vi "Actor Core.vi"(8 "error in":errorcluster, 11 "Platform in":refnum<class "Platform.lvclass">) -> (0 "error out":errorcluster, 3 "Actor out":refnum<class "Actor.lvclass">)   [LabVIEW 2019, in "Platform.lvlib" / "Platform.lvclass"]
doc: "(<B>Filename</B>: Actor Framework.lvlib:Actor.lvclass:Actor Core.vi)\n\nReceives messages to the actor, reacts to them, and initiates any error handling that may shut the actor down.\n\nDescendant classes may override this VI to append parallel tasks for the actor to complete while it handles messages. Overrides use the Call Parent Method node."
uses:
  Platform.lvclass
  C:/Program Files (x86)/National Instruments/LabVIEW 2019/vi.lib/MGI/Panel Manager/Panel Actor/Panel Actor/Panel Actor.lvclass
  C:/Program Files (x86)/National Instruments/LabVIEW 2019/vi.lib/ActorFramework/Actor/Actor.lvclass
  <vilib>/ActorFramework/Actor/Actor.lvclass
  Platform.lvclass/Platform.ctl
  <vilib>/ActorFramework/Message Enqueuer/Message Enqueuer.lvclass/Message Enqueuer.ctl
  Sequence/Sequence Messages/Load Seq Msg/Load Seq Msg.lvclass/Load Seq Msg.ctl
  Sequence/Sequence Messages/Update Seq Msg/Update Seq Msg.lvclass/Update Seq Msg.ctl
  <vilib>/ActorFramework/Actor/Actor.lvclass/Actor.ctl
  Timer/Timer Messages/Start Timer Msg/Start Timer Msg.lvclass/Start Timer Msg.ctl
  Platform Messages/Run Msg/PF Commands Msg.lvclass/PF Commands Msg.ctl
  <vilib>/ActorFramework/Message Enqueuer/Enqueue.vi
  Timer/Timer Messages/Read Timer Msg/Read Timer Msg.lvclass
  C:/Program Files (x86)/National Instruments/LabVIEW 2019/vi.lib/ActorFramework/Message/Message.lvclass
  Sequence/Sequence Messages/Load Seq Msg/Load Seq Msg.lvclass
  Sequence/Sequence Messages/Update Seq Msg/Update Seq Msg.lvclass
  Timer/Timer Messages/Pause Timer Msg/Pause Timer Msg.lvclass
  Timer/Timer Messages/Resume Timer Msg/Resume Timer Msg.lvclass
  Timer/Timer Messages/Start Timer Msg/Start Timer Msg.lvclass
  Platform Messages/Run Msg/PF Commands Msg.lvclass
  <vilib>/ActorFramework/Stop Msg/Stop Msg.lvclass
  <userlib>/_MGI/Application Control/MGI Get Value/MGI Get Value (BOOL).vi
  <userlib>/_MGI/Application Control/MGI Get Value/MGI Get Value (I32).vi
  <vilib>/ActorFramework/Message Priority Queue/Priority Enqueue.vi
  <userlib>/_MGI/Application Control/MGI Gray if/MGI Gray if False.vi
  <vilib>/MGI/Panel Manager/Panel Actor/Panel Actor/Panel Actor.lvclass
panel:
  in  "Sequence":T1(array[cluster]) {"Duration" format="%<%H:%M:%S>t"}
  in  "Clear":bool
  in  "Save":bool
  in  "Sequence File Path":path=path "C:/Working Copy/trunk/Modified Cobra Jung/Cobra/Power Pattern Configuration/TTV.ini" caption="Path"
  out "Saving":bool
  out "Mini Graph":u32[](graph)
  in  "Run":bool
  out "Current Step":i32=1 caption="Step"
  out "Current Iteration":i32=1 caption="Iteration"
  in  "Reset Test":bool
  out "Elapsed Time":dbl caption="Time(sec)" format="%<%H:%M:%S>t"
  out "Test Graph":dbl[][](graph)
  in  "Iteration":i32=2
  out "Save File Path":path caption="Path"
  # "Step"
  # "Duration"
  # "Amplitute"
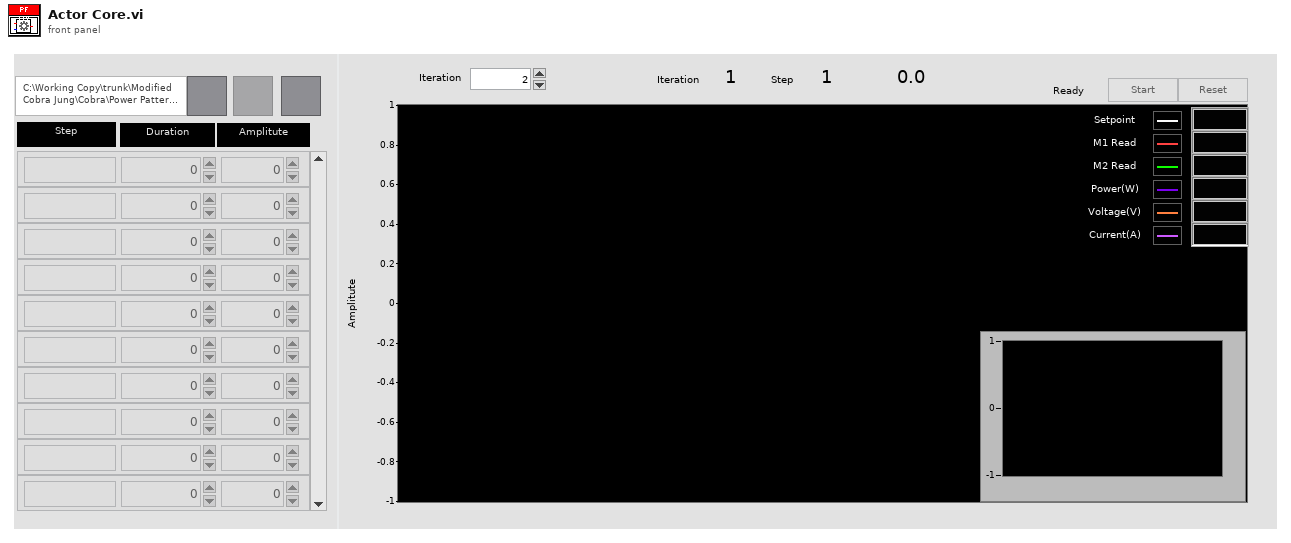
[diagram p1: front panel]
types:
  T1 = cluster{"Duration":i32, "Value":u32, "Name":string}[]
  T2 = enum32{"Invalid", "Standard", "Closed", "Hidden", "Minimized", "Maximized"}
  T3 = cluster{"Event Registration Refnum":refnum<event-registration>, "Pnl Actor":refnum<event-registration>}
  T4 = enum8{"Enabled", "Disabled", "Disabled and Grayed Out"}
  T5 = cluster{"Duration":i32, "Value":u32, "Name":string}
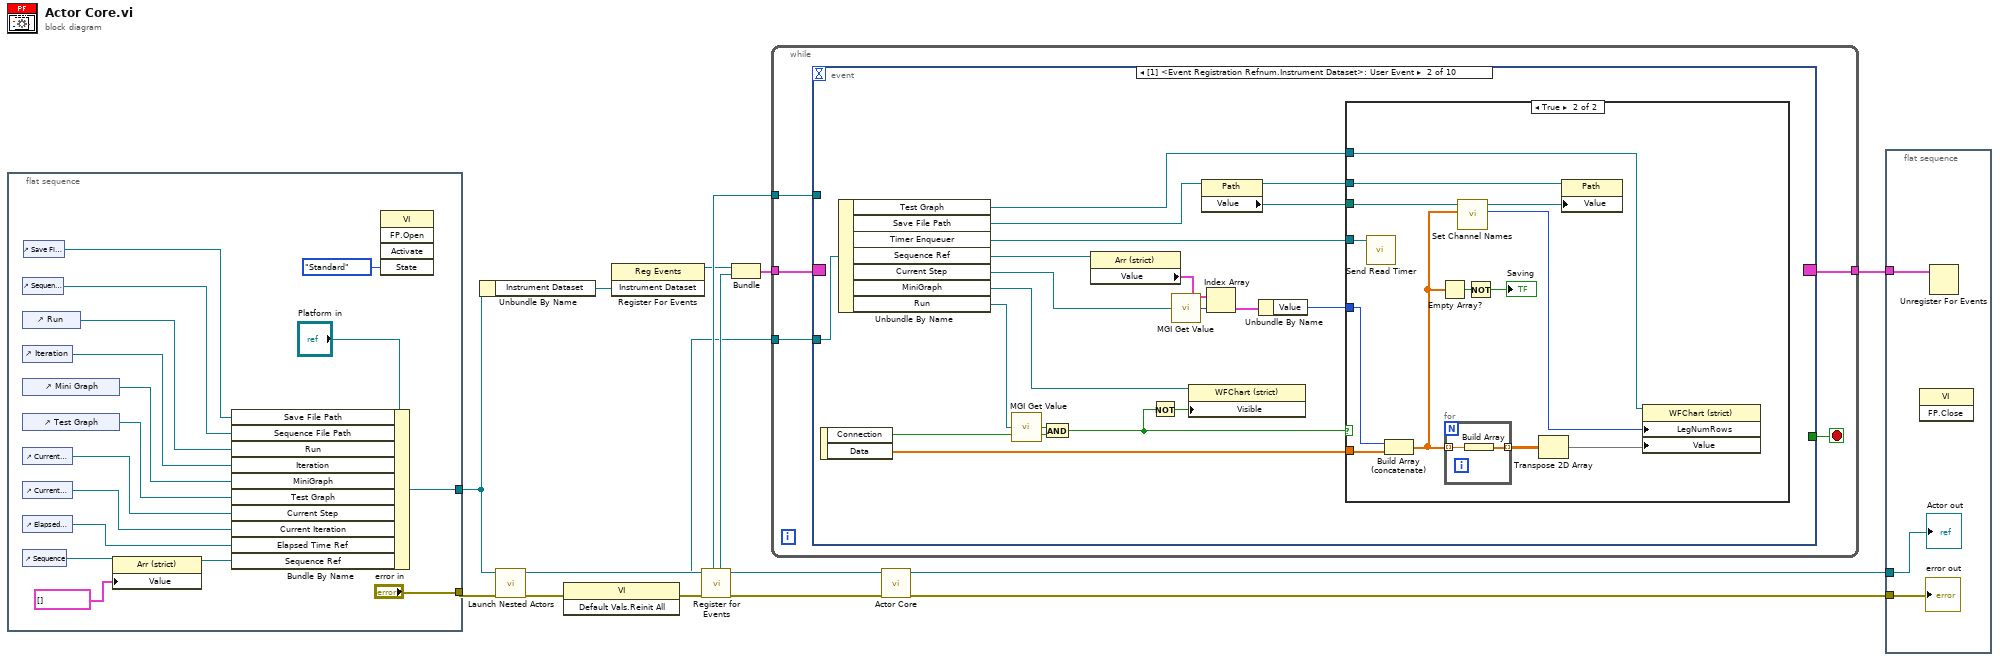
[diagram p0: block diagram]
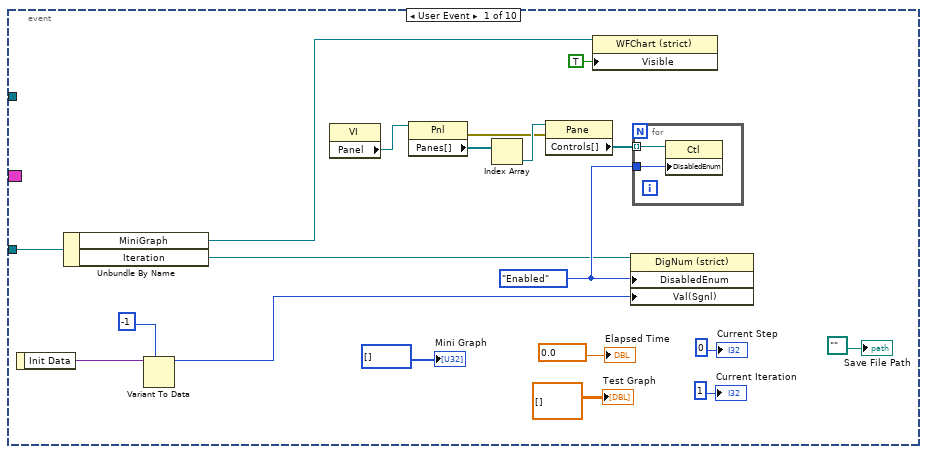
[diagram p2: hidden frame]
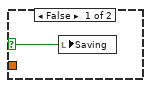
[diagram p3: hidden frame]
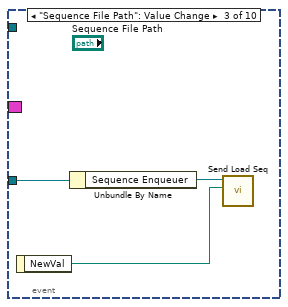
[diagram p4: hidden frame]
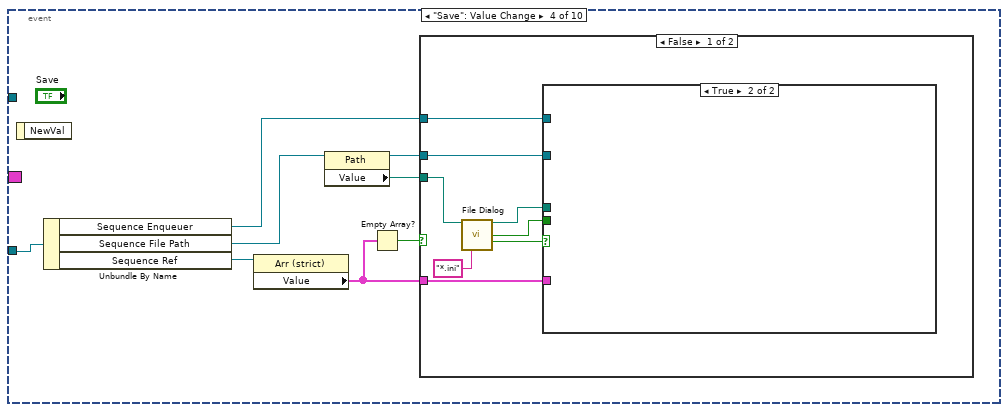
[diagram p5: hidden frame]
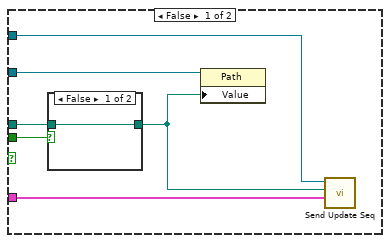
[diagram p6: hidden frame]
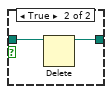
[diagram p7: hidden frame]
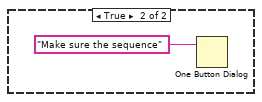
[diagram p8: hidden frame]
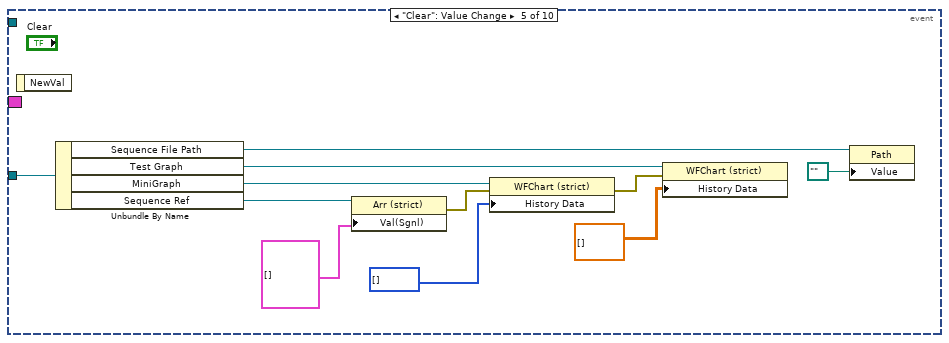
[diagram p9: hidden frame]
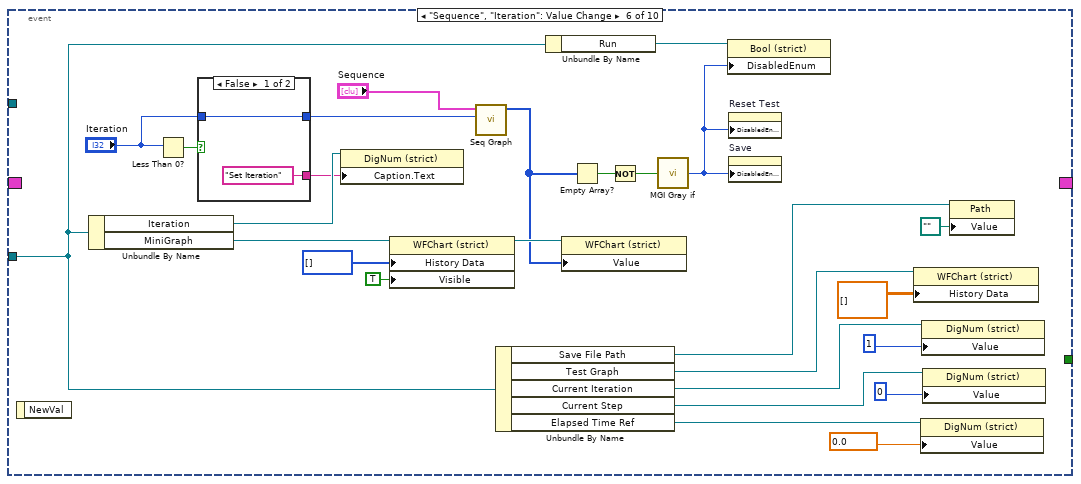
[diagram p10: hidden frame]
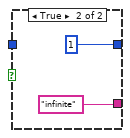
[diagram p11: hidden frame]
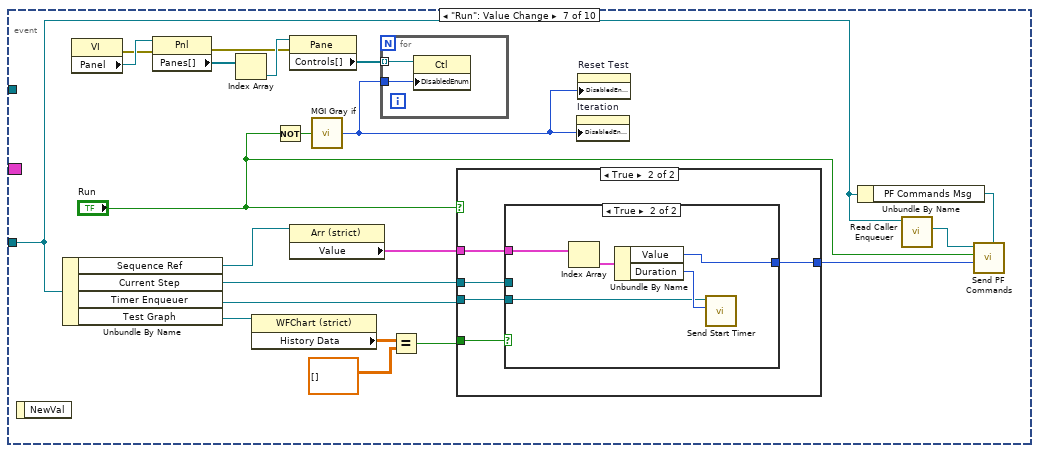
[diagram p12: hidden frame]
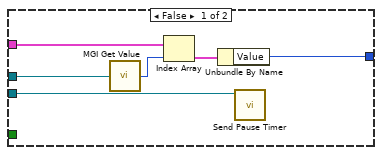
[diagram p13: hidden frame]
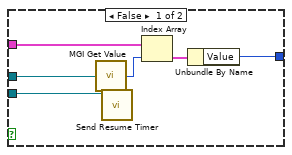
[diagram p14: hidden frame]
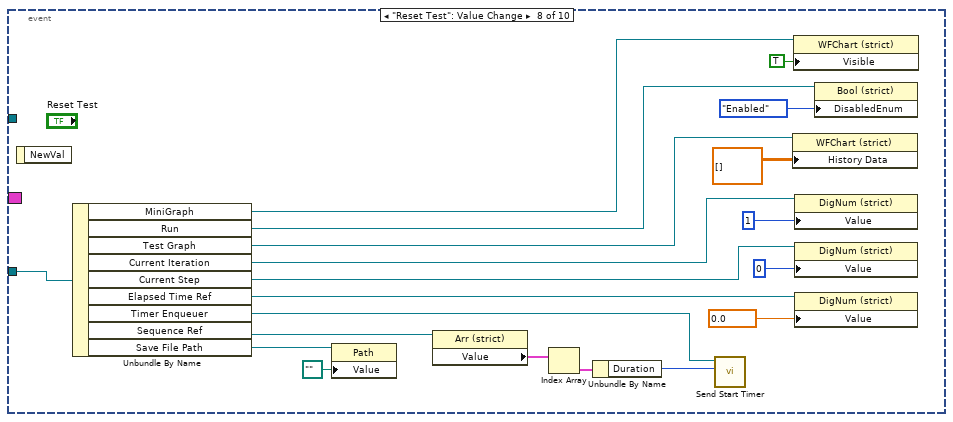
[diagram p15: hidden frame]
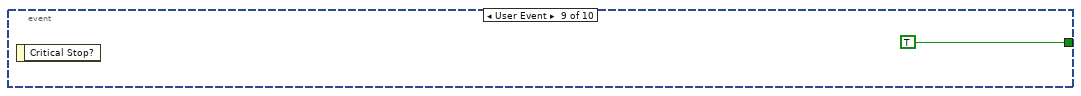
[diagram p16: hidden frame]
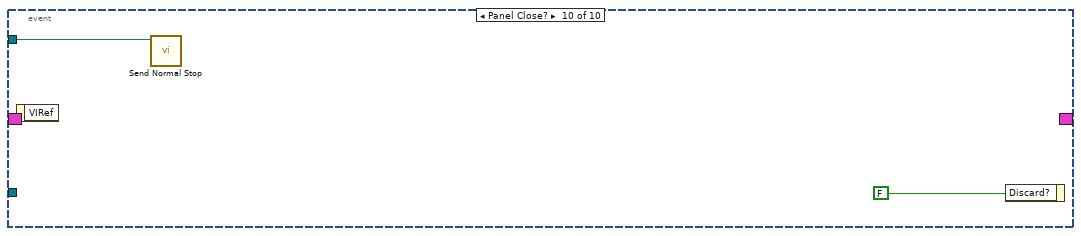
[diagram p17: hidden frame]
diagram:
  n1 = flat-sequence {
    tunnel: ["error in"] -> w5
    tunnel: [w24] -> w4
    frame #0 {
      n2 = control-ref of="Sequence File Path"() -> (w17:refnum<vi>)
      n3 = control-ref of="Run"() -> (w23:refnum<vi>)
      n4 = control-ref of="Iteration"() -> (w25:refnum<vi>)
      n5 = control-ref of="Mini Graph"() -> (w22:refnum<vi>)
      n6 = control-ref of="Test Graph"() -> (w21:refnum<vi>)
      n7 = control-ref of="Current Step"() -> (w28:refnum<vi>)
      n8 = control-ref of="Current Iteration"() -> (w27:refnum<vi>)
      n9 = control-ref of="Elapsed Time"() -> (w29:refnum<vi>)
      n10 = control-ref of="Sequence"() -> (w19:refnum<vi>)
      n11 = control-ref of="Save File Path"() -> (w16:refnum<vi>)
      n12 = property class="Arr (strict)"(reference=w19, "Value"=T1 [] ("Sequence")) -> (reference out=w18:refnum<vi>)  [unwired: 1 in, 1 out]
      n13 = Bundle By Name(cluster="Platform in", "Save File Path"=w16, "Sequence File Path"=w17, "Run"=w23, "Iteration"=w25, "MiniGraph"=w22, "Test Graph"=w21, "Current Step"=w28, "Current Iteration"=w27, "Elapsed Time Ref"=w29, "Sequence Ref"=w18) -> (w24:refnum<class "Platform.lvclass">)
      n14 = invoke class="VI" method="FP.Open"("State"=T2."Standard") -> ()  [unwired: 4 in, 5 out]
    }
  }
  n15 = Unbundle By Name(w4) -> ("Instrument Dataset"=w9:refnum<user-event>)
  n16 = call-dynamic "Launch Nested Actors.vi"("error in"=w5, "Platform in"=w4) -> ("error out"=w3:errorcluster, "Platform out"=w11:refnum<class "Platform.lvclass">)  [unwired: 8 in]
  n17 = invoke class="VI" method="Default Vals.Reinit All"(error in=w3) -> (error out=w2:errorcluster)  [unwired: 2 in, 2 out]
  n18 = register-events(w9) -> (reference out=w6:refnum<event-registration>)  [unwired: 2 in, 1 out]
  n19 = call <vilib>:"Register for Events.vi"("Error In"=w2, "Panel Actor in"=w11) -> ("Error Out"=w12:errorcluster, "Panel Actor out"=w1:refnum<class "Platform.lvclass">, "Pnl Actor"=w8:refnum<event-registration>, "Self Enqueuer"=w10:refnum<class "Message Enqueuer.lvclass">)  [unwired: 6 in]
  n20 = Bundle("Event Registration Refnum"=w6, "Pnl Actor"=w8) -> (w7:T3)  [unwired: 1 in]
  n21 = while {
    tunnel: w7 -> [w36]
    tunnel: [w34] -> w13
    tunnel: w10 -> [w33]
    tunnel: w1 -> [w32]
    stop <- w35 stop-if-true
    n22 = event shown="[1] <Event Registration Refnum.Instrument Dataset>: User Event" {
      selector: w36 -> [_ _ _ _ _ _ _ _ _ _]
      dyn-events: [_ _ _ _ _ _ _ _ _ _] -> w34
      timeout: _ -> [_ _ _ _ _ _ _ _ _ _]
      tunnel: [_ _ _ _ _ _ _ _ TRUE _] -> w35
      tunnel: w33 -> [_ _ _ _ _ _ _ _ _ w229]
      tunnel: w32 -> [w54 w73 w94 w103 w132 w143 w167 w225 _ _]
      event User Event {
        w47 = T4."Enabled" ("Disabled")
        n23 = event-data() -> ("Init Data"=w55:variant)  [unwired: 1 in]
        n24 = Unbundle By Name(w54) -> ("MiniGraph"=w44:refnum<vi>, "Iteration"=w46:refnum<vi>)
        n25 = Variant To Data(type=-1 ("Value (Signaling)"), Variant=w55) -> (data=w37:i32)  [unwired: 1 in, 1 out]
        n26 = property class="VI"() -> ("Panel"=w48:refnum<vi>)  [unwired: 2 in, 2 out]
        n27 = property class="Pnl"(reference=w48) -> (error out=w49:errorcluster, "Panes[]"=w52:refnum<vi>[])  [unwired: 1 in, 1 out]
        n28 = Index Array(array=w52) -> (element=w51:refnum<vi>)  [unwired: 1 in]
        n29 = property class="Pane"(reference=w51, error in=w49) -> ("Controls[]"=w50:refnum<vi>[])  [unwired: 2 out]
        n30 = property class="WFChart (strict)"(reference=w44, "Visible"=TRUE) -> ()  [unwired: 1 in, 2 out]
        n31 = property class="DigNum (strict)"(reference=w46, "DisabledEnum"=w47, "Val(Sgnl)"=w37) -> ()  [unwired: 1 in, 2 out]
        n32 = for {
          tunnel: w50 -> [w57] mode=indexing
          tunnel: w47 -> [w56]
          n33 = property class="Ctl"(reference=w57, "DisabledEnum"=w56) -> ()  [unwired: 1 in, 2 out]
        }
        "Current Step" <- 0 ("Current Step")
        "Current Iteration" <- 1 ("Current Iteration")
        "Mini Graph" <- u32[] [] ("Test Graph")
        "Elapsed Time" <- 0.0 ("Time")
        "Test Graph" <- dbl[][] [] ("Test Graph")
        "Save File Path" <- path "" ("Save File Path")
      }
      event User Event {
        n34 = event-data() -> ("Connection"=w68:bool, "Data"=w76:dbl[])  [unwired: 1 in]
        n35 = Unbundle By Name(w73) -> ("Test Graph"=w58:refnum<vi>, "Save File Path"=w63:refnum<vi>, "Timer Enqueuer"=w67:refnum<class "Message Enqueuer.lvclass">, "Sequence Ref"=w75:refnum<vi>, "Current Step"=w72:refnum<vi>, "MiniGraph"=w61:refnum<vi>, "Run"=w64:refnum<vi>)
        n36 = call-poly <userlib>:"MGI Get Value.vi"("Ref"=w64) -> ("Value"=w65:bool)
        n37 = And(x=w65, y=w68) -> (x .and. y?=w60:bool)
        n38 = property class="Arr (strict)"(reference=w75) -> ("Value"=w74:T1)  [unwired: 1 in, 2 out]
        n39 = Not(x=w60) -> (.not. x?=w66:bool)
        n40 = call-poly <userlib>:"MGI Get Value.vi"("Ref"=w72) -> ("Value"=w71:i32)
        n41 = property class="WFChart (strict)"(reference=w61, "Visible"=w66) -> ()  [unwired: 1 in, 2 out]
        n42 = property class="Path"(reference=w63) -> (reference out=w59:refnum<vi>, "Value"=w62:path)  [unwired: 1 in, 1 out]
        n43 = Index Array(array=w74, index=w71) -> (element=w70:T5)
        n44 = Unbundle By Name(w70) -> ("Value"=w69:u32)
        n45 = case shown="True" w60 {
          selector: w60 -> [w77 _]
          tunnel: w76 -> [_ w80]
          tunnel: w67 -> [_ w90]
          tunnel: w69 -> [_ w81]
          tunnel: w62 -> [_ w85]
          tunnel: w59 -> [_ w89]
          tunnel: w58 -> [_ w87]
          frame False {
            n46 = local write "Saving"(w77) -> ()
          }
          frame True {
            n47 = call "Send Read Timer.vi"("Message Enqueuer"=w90) -> ()  [unwired: 9 in, 2 out]
            n48 = Build Array (concatenate)(w81, w80) -> (w79:dbl[])
            n49 = Empty Array?(array=w79) -> (empty?=w88:bool)
            n50 = for {
              tunnel: w79 -> [w91] mode=indexing
              tunnel: [w92] -> w86 mode=indexing
              n51 = Build Array(w91) -> (w92:dbl[])
            }
            n52 = call "Set Channel Names.vi"("Data"=w79, "file path (dialog if empty)"=w85) -> ("Channel Length"=w83:i32, "new file path (Not A Path if cancelled)"=w84:path)  [unwired: 8 in]
            n53 = Not(x=w88) -> (.not. x?=→"Saving":bool)
            n54 = Transpose 2D Array(2D array=w86) -> (transposed array=w82:dbl[][])
            n55 = property class="Path"(reference=w89, "Value"=w84) -> ()  [unwired: 1 in, 2 out]
            n56 = property class="WFChart (strict)"(reference=w87, "LegNumRows"=w83, "Value"=w82) -> ()  [unwired: 1 in, 2 out]
          }
        }
      }
      event "Sequence File Path": Value Change {
        n57 = event-data() -> ("NewVal"=w95:path)  [unwired: 1 in]
        n58 = Unbundle By Name(w94) -> ("Sequence Enqueuer"=w93:refnum<class "Message Enqueuer.lvclass">)
        n59 = call "Send Load Seq.vi"("Seq file path"=w95, "Message Enqueuer"=w93) -> ()  [unwired: 8 in, 2 out]
      }
      event "Save": Value Change {
        n60 = event-data() -> ()  [unwired: 1 in, 1 out]
        n61 = Unbundle By Name(w103) -> ("Sequence Enqueuer"=w97:refnum<class "Message Enqueuer.lvclass">, "Sequence File Path"=w99:refnum<vi>, "Sequence Ref"=w102:refnum<vi>)
        n62 = property class="Arr (strict)"(reference=w102) -> ("Value"=w101:T1)  [unwired: 1 in, 2 out]
        n63 = property class="Path"(reference=w99) -> (reference out=w96:refnum<vi>, "Value"=w98:path)  [unwired: 1 in, 1 out]
        n64 = Empty Array?(array=w101) -> (empty?=w100:bool)
        n65 = case shown="False" w100 {
          tunnel: w97 -> [w107 _]
          tunnel: w101 -> [w106 _]
          tunnel: w98 -> [w111 _]
          tunnel: w96 -> [w104 _]
          frame False {
            n66 = call "File Dialog"("start path"=w111, "pattern (all files)"="*.ini") -> ("selected path"=w108:path, "exists"=w109:bool, "cancelled"=w105:bool)  [unwired: 10 in, 1 out]
            n67 = case shown="True" w105 {
              tunnel: w109 -> [w117 _]
              tunnel: w108 -> [w116 _]
              tunnel: w107 -> [w115 _]
              tunnel: w106 -> [w114 _]
              tunnel: w104 -> [w112 _]
              frame False {
                n68 = case shown="False" w117 {
                  tunnel: w116 -> [w118 w120]
                  tunnel: [w118 w119] -> w113
                  frame False {
                  }
                  frame True {
                    n69 = Delete(path (use dialog)=w120) -> (deleted path=w119:path)  [unwired: 4 in, 2 out]
                  }
                }
                n70 = property class="Path"(reference=w112, "Value"=w113) -> ()  [unwired: 1 in, 2 out]
                n71 = call "Send Update Seq.vi"("Sequence"=w114, "file path"=w113, "Message Enqueuer"=w115) -> ()  [unwired: 7 in, 2 out]
              }
              frame True {
              }
            }
          }
          frame True {
            n72 = One Button Dialog(message="Make sure the sequence") -> ()  [unwired: 1 in, 1 out]
          }
        }
      }
      event "Clear": Value Change {
        n73 = event-data() -> ()  [unwired: 1 in, 1 out]
        n74 = Unbundle By Name(w132) -> ("Sequence File Path"=w123:refnum<vi>, "Test Graph"=w131:refnum<vi>, "MiniGraph"=w130:refnum<vi>, "Sequence Ref"=w128:refnum<vi>)
        n75 = property class="Arr (strict)"(reference=w128, "Val(Sgnl)"=T1 [] ("Value (Signaling)")) -> (error out=w126:errorcluster)  [unwired: 1 in, 1 out]
        n76 = property class="WFChart (strict)"(reference=w130, error in=w126, "History Data"=u32[] []) -> (error out=w125:errorcluster)  [unwired: 1 out]
        n77 = property class="WFChart (strict)"(reference=w131, error in=w125, "History Data"=dbl[][] [] ("Test Graph")) -> ()  [unwired: 2 out]
        n78 = property class="Path"(reference=w123, "Value"=path "" ("Sequence File Path")) -> ()  [unwired: 1 in, 2 out]
      }
      event "Sequence", "Iteration": Value Change {
        n79 = event-data() -> ()  [unwired: 1 in, 1 out]
        n80 = Unbundle By Name(w143) -> ("Iteration"=w151:refnum<vi>, "MiniGraph"=w154:refnum<vi>)
        n81 = Less Than 0?(x="Iteration") -> (x < 0?=w156:bool)
        n82 = case shown="False" w156 {
          tunnel: "Iteration" -> [w160 _]
          tunnel: [w160 1 ("t")] -> w157
          tunnel: ["Set Iteration" ("Inifinite") "infinite" ("Inifinite")] -> w150
          frame False {
          }
          frame True {
          }
        }
        n83 = property class="DigNum (strict)"(reference=w151, "Caption.Text"=w150) -> ()  [unwired: 1 in, 2 out]
        n84 = property class="WFChart (strict)"(reference=w154, "History Data"=u32[] [], "Visible"=TRUE) -> (reference out=w152:refnum<vi>)  [unwired: 1 in, 1 out]
        n85 = call "Seq Graph.vi"("Iteration"=w157, "Sequence"="Sequence") -> ("Waveform"=w141:u32[])  [unwired: 8 in, 1 out]
        n86 = Unbundle By Name(w143) -> ("Save File Path"=w134:refnum<vi>, "Test Graph"=w140:refnum<vi>, "Current Iteration"=w147:refnum<vi>, "Current Step"=w148:refnum<vi>, "Elapsed Time Ref"=w149:refnum<vi>)
        n87 = Unbundle By Name(w143) -> ("Run"=w142:refnum<vi>)
        n88 = property class="WFChart (strict)"(reference=w152, "Value"=w141) -> ()  [unwired: 1 in, 2 out]
        n89 = Empty Array?(array=w141) -> (empty?=w138:bool)
        n90 = Not(x=w138) -> (.not. x?=w137:bool)
        n91 = call-poly <userlib>:"MGI Gray if.vi"("Boolean"=w137) -> ("Disabled"=w136:T4)
        n92 = property class="Bool (strict)"(reference=w142, "DisabledEnum"=w136) -> ()  [unwired: 1 in, 2 out]
        n93 = property on="Reset Test" class="Bool"("DisabledEnum"=w136) -> ()  [unwired: 2 in, 2 out]
        n94 = property on="Save" class="Bool"("DisabledEnum"=w136) -> ()  [unwired: 2 in, 2 out]
        n95 = property class="WFChart (strict)"(reference=w140, "History Data"=dbl[][] [] ("Test Graph")) -> ()  [unwired: 1 in, 2 out]
        n96 = property class="DigNum (strict)"(reference=w149, "Value"=0.0 ("Time")) -> ()  [unwired: 1 in, 2 out]
        n97 = property class="DigNum (strict)"(reference=w147, "Value"=1) -> ()  [unwired: 1 in, 2 out]
        n98 = property class="DigNum (strict)"(reference=w148, "Value"=0) -> ()  [unwired: 1 in, 2 out]
        n99 = property class="Path"(reference=w134, "Value"=path "") -> ()  [unwired: 1 in, 2 out]
      }
      event "Run": Value Change {
        n100 = event-data() -> ()  [unwired: 1 in, 1 out]
        n101 = Unbundle By Name(w167) -> ("Sequence Ref"=w168:refnum<vi>, "Current Step"=w172:refnum<vi>, "Timer Enqueuer"=w183:refnum<class "Message Enqueuer.lvclass">, "Test Graph"=w171:refnum<vi>)
        n102 = property class="VI"() -> (error out=w178:errorcluster, "Panel"=w182:refnum<vi>)  [unwired: 2 in, 1 out]
        n103 = property class="Pnl"(reference=w182, error in=w178) -> (error out=w177:errorcluster, "Panes[]"=w181:refnum<vi>[])  [unwired: 1 out]
        n104 = Index Array(array=w181) -> (element=w180:refnum<vi>)  [unwired: 1 in]
        n105 = property class="WFChart (strict)"(reference=w171) -> ("History Data"=w170:dbl[][])  [unwired: 1 in, 2 out]
        n106 = Not(x="Run") -> (.not. x?=w165:bool)
        n107 = property class="Pane"(reference=w180, error in=w177) -> ("Controls[]"=w179:refnum<vi>[])  [unwired: 2 out]
        n108 = property class="Arr (strict)"(reference=w168) -> ("Value"=w176:T1)  [unwired: 1 in, 2 out]
        n109 = call-poly <userlib>:"MGI Gray if.vi"("Boolean"=w165) -> ("Disabled"=w164:T4)
        n110 = for {
          tunnel: w179 -> [w185] mode=indexing
          tunnel: w164 -> [w184]
          n111 = property class="Ctl"(reference=w185, "DisabledEnum"=w184) -> ()  [unwired: 1 in, 2 out]
        }
        n112 = Equal?(x=w170, y=dbl[][] [] ("Test Graph")) -> (x = y?=w166:bool)
        n113 = case shown="True" "Run" {
          tunnel: w183 -> [w191 w196]
          tunnel: w176 -> [w189 w195]
          tunnel: [w188 w194] -> w174
          tunnel: w172 -> [w187 w193]
          tunnel: w166 -> [_ w192]
          frame False {
            n114 = call-poly <userlib>:"MGI Get Value.vi"("Ref"=w187) -> ("Value"=w186:i32)
            n115 = Index Array(array=w189, index=w186) -> (element=w190:T5)
            n116 = Unbundle By Name(w190) -> ("Value"=w188:u32)
            n117 = call "Send Pause Timer.vi"("Message Enqueuer"=w191) -> ()  [unwired: 9 in, 2 out]
          }
          frame True {
            n118 = case shown="True" w192 {
              tunnel: w196 -> [w202 w204]
              tunnel: w195 -> [w200 w206]
              tunnel: [w199 w203] -> w194
              tunnel: w193 -> [w198 _]
              frame False {
                n119 = call-poly <userlib>:"MGI Get Value.vi"("Ref"=w198) -> ("Value"=w197:i32)
                n120 = call "Send Resume Timer.vi"("Message Enqueuer"=w202) -> ()  [unwired: 9 in, 2 out]
                n121 = Index Array(array=w200, index=w197) -> (element=w201:T5)
                n122 = Unbundle By Name(w201) -> ("Value"=w199:u32)
              }
              frame True {
                n123 = Index Array(array=w206) -> (element=w207:T5)  [unwired: 1 in]
                n124 = Unbundle By Name(w207) -> ("Value"=w203:u32, "Duration"=w205:i32)
                n125 = call "Send Start Timer.vi"("Time Target (s)"=w205, "Message Enqueuer"=w204) -> ()  [unwired: 8 in, 2 out]
              }
            }
          }
        }
        n126 = property on="Iteration" class="DigNum (strict)"("DisabledEnum"=w164) -> ()  [unwired: 2 in, 2 out]
        n127 = property on="Reset Test" class="Bool"("DisabledEnum"=w164) -> ()  [unwired: 2 in, 2 out]
        n128 = Unbundle By Name(w167) -> ("PF Commands Msg"=w173:refnum<class "PF Commands Msg.lvclass">)
        n129 = call <vilib>:"Read Caller Enqueuer.vi"("Actor"=w167) -> ("Caller Enqueuer"=w175:refnum<class "Message Enqueuer.lvclass">)  [unwired: 10 in]
        n130 = call "Send PF Commands.vi"("Message Type"=w173, "Setpoint"=w174, "Run"="Run", "Message Enqueuer"=w175) -> ()  [unwired: 6 in, 2 out]
      }
      event "Reset Test": Value Change {
        n131 = event-data() -> ()  [unwired: 1 in, 1 out]
        n132 = Unbundle By Name(w225) -> ("MiniGraph"=w210:refnum<vi>, "Run"=w219:refnum<vi>, "Test Graph"=w220:refnum<vi>, "Current Iteration"=w221:refnum<vi>, "Current Step"=w222:refnum<vi>, "Elapsed Time Ref"=w227:refnum<vi>, "Timer Enqueuer"=w213:refnum<class "Message Enqueuer.lvclass">, "Sequence Ref"=w217:refnum<vi>, "Save File Path"=w208:refnum<vi>)
        n133 = property class="Path"(reference=w208, "Value"=path "") -> ()  [unwired: 1 in, 2 out]
        n134 = property class="Arr (strict)"(reference=w217) -> ("Value"=w215:T1)  [unwired: 1 in, 2 out]
        n135 = Index Array(array=w215) -> (element=w216:T5)  [unwired: 1 in]
        n136 = Unbundle By Name(w216) -> ("Duration"=w214:i32)
        n137 = call "Send Start Timer.vi"("Time Target (s)"=w214, "Message Enqueuer"=w213) -> ()  [unwired: 8 in, 2 out]
        n138 = property class="WFChart (strict)"(reference=w220, "History Data"=dbl[][] [] ("Test Graph")) -> ()  [unwired: 1 in, 2 out]
        n139 = property class="WFChart (strict)"(reference=w210, "Visible"=TRUE) -> ()  [unwired: 1 in, 2 out]
        n140 = property class="DigNum (strict)"(reference=w221, "Value"=1) -> ()  [unwired: 1 in, 2 out]
        n141 = property class="DigNum (strict)"(reference=w222, "Value"=0) -> ()  [unwired: 1 in, 2 out]
        n142 = property class="DigNum (strict)"(reference=w227, "Value"=0.0 ("Time")) -> ()  [unwired: 1 in, 2 out]
        n143 = property class="Bool (strict)"(reference=w219, "DisabledEnum"=T4."Enabled" ("Disabled")) -> ()  [unwired: 1 in, 2 out]
      }
      event User Event {
        n144 = event-data() -> ()  [unwired: 1 in, 1 out]
      }
      event Panel Close? {
        n145 = event-data() -> ()  [unwired: 1 in, 1 out]
        n146 = call <vilib>:"Send Normal Stop.vi"("Message Enqueuer"=w229) -> ()  [unwired: 10 in, 1 out]
        n147 = event-data("Discard?"=FALSE) -> ()  [unwired: 1 in, 1 out]
      }
    }
  }
  n148 = call-parent "Actor Core.vi"("error in"=w12, "Panel Actor in"=w1) -> ("error out"=w15:errorcluster, "Actor out"=w14:refnum<class "Actor.lvclass">)  [unwired: 8 in]
  n149 = flat-sequence {
    tunnel: w15 -> [w233]
    tunnel: w14 -> [w232]
    tunnel: w13 -> [w231]
    frame #0 {
      n150 = invoke class="VI" method="FP.Close"() -> ()  [unwired: 3 in, 3 out]
      n151 = Unregister For Events(event registration refnum=w231) -> ()  [unwired: 1 in, 1 out]
      "error out" <- w233
      "Actor out" <- w232
    }
  }
